vi "Inverse Dynamics.vi"   [LabVIEW 2017, in "NI_Kinematics.lvlib"]
doc: "Returns the amount of torque required for the robotic arm to achieve the joint positions, velocities, and accelerations you specify. Wire data to the <B>joint positions</B> input to determine the polymorphic instance to use or manually select the instance.\n\n<B>.m file:</B> rne"
uses:
  <vilib>/robotics/Kinematics/NI_Kinematics.lvlib
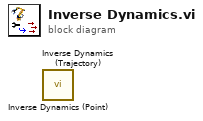
[diagram p0: block diagram]
diagram:
  n1 = call <vilib>:"Inverse Dynamics (Point).vi"() -> ()  [unwired: 13 in, 3 out]
  n2 = call <vilib>:"Inverse Dynamics (Trajectory).vi"() -> ()  [unwired: 13 in, 3 out]
